vi "vi_out.vi"(0 "Numeric Control":dbl, 1 "Numeric":dbl, 2 "Array - String":string[](array[string]), 3 "Real Matrix":dbl[][](array[numeric]), 4 "OK Button":bool, 5 "Vertical Fill Slide":dbl(slide) scale=0.0..10.0, 6 "Pict Ring":u16(ring), 7 "Digital Data":digitaldata, 8 "Knob":dbl(knob) scale=0.0..10.0, 9 "Color Box":u32(colorbox), 10 "Listbox":i32(listbox)=1, 11 "Waveform":waveform(dbl), 12 "Cluster":T1={"Cluster"={"Cluster"={"Cluster"={"Time Stamp Control"=timestamp(3385069200 s since 1904-01-01), "Array - Numeric"=[1.0, 2.0, 3.0]}, "OK Button 2"=TRUE, "Cancel Button"=FALSE}, "Array - String"=["magus", "francisco"]}, "Listbox"=1}, 13 "Waveform Chart":dbl(graph), 14 "Boolean":bool, 15 "Boolean 2":bool, 16 "String":string, 17 "Combo Box":string(combo), 18 "Waveform Graph":dbl[](graph), 19 "XY Graph":cluster{dbl, dbl}[](graph), 20 "Enum":enum16{""}(ring), 21 "File Path Control":path, 24 "Array":dbl[](array[numeric]), 25 "Array - Numeric":dbl[](array[numeric]), 27 "Text Ring":u16(ring)) -> ()   [LabVIEW 2011]
panel:
  in  "stop":bool
  in  "Error In":errorcluster
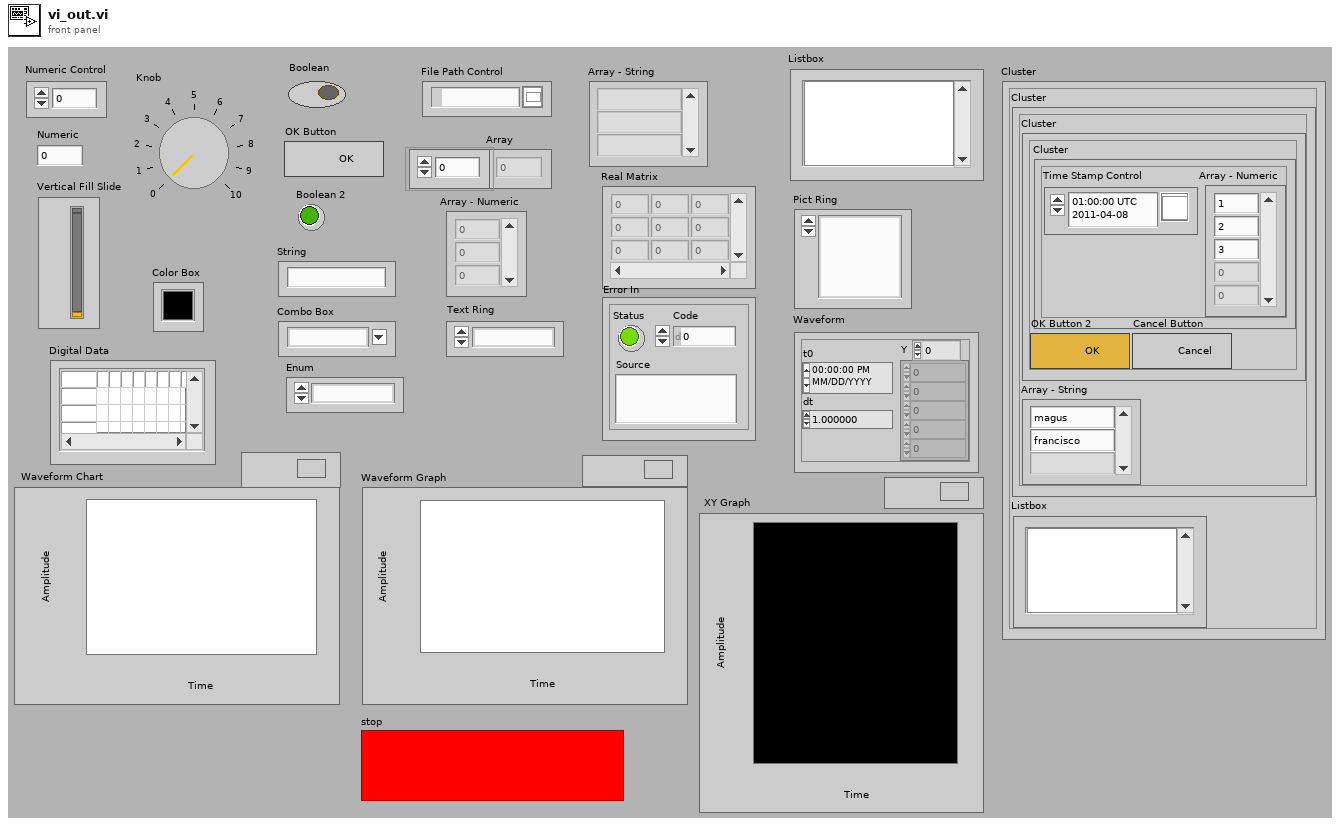
[diagram p1: front panel]
types:
  T1 = cluster{"Cluster":cluster{"Cluster":cluster{"Cluster":cluster{"Time Stamp Control":timestamp, "Array - Numeric":dbl[]}, "OK Button 2":bool, "Cancel Button":bool}, "Array - String":string[]}, "Listbox":i32}
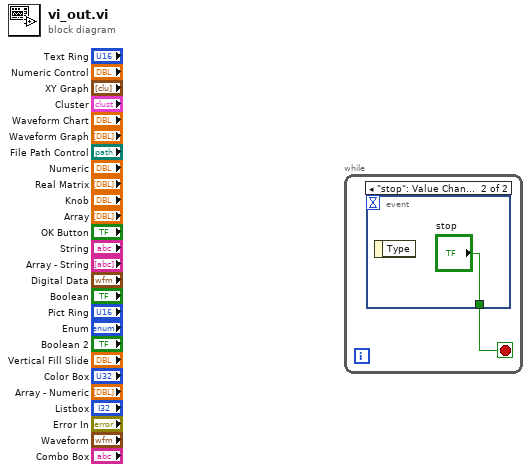
[diagram p0: block diagram]
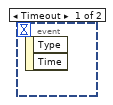
[diagram p2: hidden frame]
diagram:
  n1 = while {
    stop <- w1 stop-if-true
    n2 = event shown="[1] \"stop\": Value Change" {
      selector: _ -> [_ _]
      dyn-events: _ -> [_ _]
      timeout: _ -> [_ _]
      tunnel: [_ "stop"] -> w1
      event Timeout {
        n3 = event-data() -> ()  [unwired: 1 in, 2 out]
      }
      event "stop": Value Change {
        n4 = event-data() -> ()  [unwired: 1 in, 1 out]
      }
    }
  }
